vi "initialize Session Data.vi"(0 "Session in":refnum<class "TestDataMgr.lvclass">, 11 "error in":errorcluster) -> (4 "Session out":refnum<class "TestDataMgr.lvclass">, 15 "error out":errorcluster)   [LabVIEW 2018, in "TestDataMgr.lvclass"]
uses:
  TestDataMgr.lvclass
  Typedefs/Test Data All.ctl
  Typedefs/Test Limits.ctl
  Typedefs/Test Raw Data.ctl
  TestDataMgr.lvclass/TestDataMgr.ctl
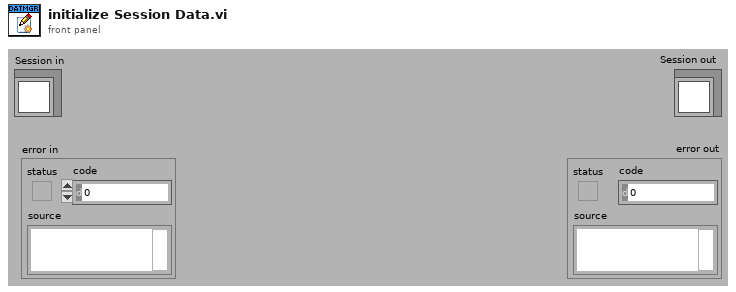
[diagram p1: front panel]
types:
  T1 = typedef "TestDataMgr.lvclass/Test Data All.ctl" = cluster{"Test Name":string, "Test Limits":T2, "Raw Data Per Tester":T3[]}
  T2 = typedef "TestDataMgr.lvclass/Test Limits.ctl" = cluster{"High":dbl, "Low":dbl}
  T3 = typedef "TestDataMgr.lvclass/Test Raw Data.ctl" = cluster{"Data":dbl[][], "Tester#":u8}
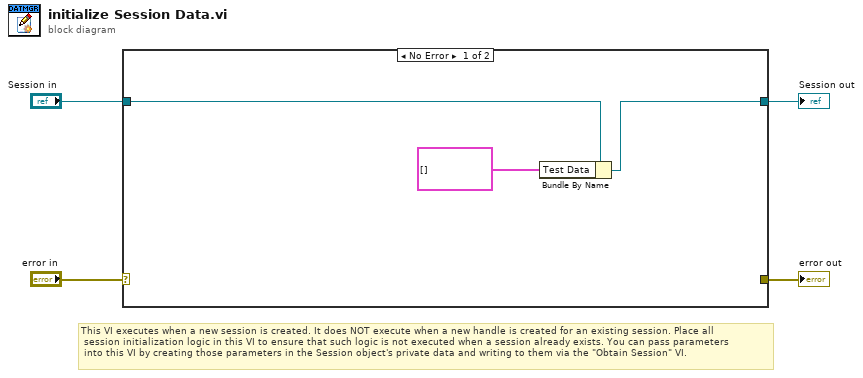
[diagram p0: block diagram]
diagram:
  # "This VI executes when a new session is created. It does NOT execute when a new handle is created for an existing session. Place all\n session initialization logic in this VI to ensure that such logic is not executed when a session already exists. You can pass parameters\n into this VI by creating those parameters in the Session object's private data and writing to them via the \"Obtain Session\" VI."
  n1 = case shown="No Error" "error in" {
    selector: "error in" -> [_ w8]
    tunnel: "Session in" -> [w5 w9]
    tunnel: [w7 w9] -> w2
    tunnel: [_ w8] -> w1
    frame No Error {
      n2 = Bundle By Name(cluster=w5, "Test Data"=T1[] []) -> (w7:refnum<class "TestDataMgr.lvclass">)
    }
    frame Error {
    }
  }
  "error out" <- w1
  "Session out" <- w2
